vi "Screw.vi"(10 "Clibration 2":T13={"cam 0"={"incident ANGLE COMPENSATION"=[], "dp/B [MeV/C/B]"=[], "charge compensation"=[], "Momentum [MeV/C]"=[], "energyDependence Input"=[], "pixel angle (y)"=[], "dp [MeV/C/] "=[], "angle 2Dfor spectrumj"=[], "dp [MeV/C] 2D"=[], "charge compensation 2D"=[], "Screen&Camera 2"={"Screen Orientation"="Regular", "Screen angle"="Flat", "Lens"=enum."FL1-f8x08", "Calibration (mm/pix)"=1.0}, "ROI info"={"npix-X"=0, "npix-Y"=0, "Left [pix]"=0.0, "Top [pix]"=0.0}, "Y 2D full angle"=[], "calib pixel"={"y1(pixel)"=[], "y2(pixel)"=[], "dp/B [MeV/C/B] (pixel)"=[], "energyDependence Input(pixel)"=[], "bending angle [deg](pixel)"=[], "total path(pixel)"=[], "pixel angle (y)(pixel)"=[], "energy dependence (pixel)"=[], "charge compensation (pixel)"=[], "Momentum [MeV/C](pixel)"=[], "angular compensation(pixel)"=[]}, "2D"={"dp"=[], "chargeCompensation"=[], "angle"=[], "Momentum"=[]}, "UserROI"={"Width"=0.0, "Hight"=0.0, "OffsetX"=0.0, "OffsetY"=0.0}, "final"={"X"=[], "xi"=[], "delta momentum"=0.0, "Y"=[], "yi"=[], "angle (Y)"=[], "delta angle"=0.0, "scale delta angle"=0.0, "intraX"=0.0, "intraY"=0.0, "mask"=[]}, "B[T]"=0.0, "index"=0.0}, "cam 1"={"incident ANGLE COMPENSATION"=[], "dp/B [MeV/C/B]"=[], "charge compensation"=[], "Momentum [MeV/C]"=[], "energyDependence Input"=[], "pixel angle (y)"=[], "dp [MeV/C/] "=[], "angle 2Dfor spectrumj"=[], "dp [MeV/C] 2D"=[], "charge compensation 2D"=[], "Screen&Camera 2"={"Screen Orientation"="Regular", "Screen angle"="Flat", "Lens"=enum."FL1-f8x08", "Calibration (mm/pix)"=1.0}, "ROI info"={"npix-X"=0, "npix-Y"=0, "Left [pix]"=0.0, "Top [pix]"=0.0}, "Y 2D full angle"=[], "calib pixel"={"y1(pixel)"=[], "y2(pixel)"=[], "dp/B [MeV/C/B] (pixel)"=[], "energyDependence Input(pixel)"=[], "bending angle [deg](pixel)"=[], "total path(pixel)"=[], "pixel angle (y)(pixel)"=[], "energy dependence (pixel)"=[], "charge compensation (pixel)"=[], "Momentum [MeV/C](pixel)"=[], "angular compensation(pixel)"=[]}, "2D"={"dp"=[], "chargeCompensation"=[], "angle"=[], "Momentum"=[]}, "UserROI"={"Width"=0.0, "Hight"=0.0, "OffsetX"=0.0, "OffsetY"=0.0}, "final"={"X"=[], "xi"=[], "delta momentum"=0.0, "Y"=[], "yi"=[], "angle (Y)"=[], "delta angle"=0.0, "scale delta angle"=0.0, "intraX"=0.0, "intraY"=0.0, "mask"=[]}, "B[T]"=0.0, "index"=0.0}, "cam 2"={"incident ANGLE COMPENSATION"=[], "dp/B [MeV/C/B]"=[], "charge compensation"=[], "Momentum [MeV/C]"=[], "energyDependence Input"=[], "pixel angle (y)"=[], "dp [MeV/C/] "=[], "angle 2Dfor spectrumj"=[], "dp [MeV/C] 2D"=[], "charge compensation 2D"=[], "Screen&Camera 2"={"Screen Orientation"="Regular", "Screen angle"="Flat", "Lens"=enum."FL1-f8x08", "Calibration (mm/pix)"=1.0}, "ROI info"={"npix-X"=0, "npix-Y"=0, "Left [pix]"=0.0, "Top [pix]"=0.0}, "Y 2D full angle"=[], "calib pixel"={"y1(pixel)"=[], "y2(pixel)"=[], "dp/B [MeV/C/B] (pixel)"=[], "energyDependence Input(pixel)"=[], "bending angle [deg](pixel)"=[], "total path(pixel)"=[], "pixel angle (y)(pixel)"=[], "energy dependence (pixel)"=[], "charge compensation (pixel)"=[], "Momentum [MeV/C](pixel)"=[], "angular compensation(pixel)"=[]}, "2D"={"dp"=[], "chargeCompensation"=[], "angle"=[], "Momentum"=[]}, "UserROI"={"Width"=0.0, "Hight"=0.0, "OffsetX"=0.0, "OffsetY"=0.0}, "final"={"X"=[], "xi"=[], "delta momentum"=0.0, "Y"=[], "yi"=[], "angle (Y)"=[], "delta angle"=0.0, "scale delta angle"=0.0, "intraX"=0.0, "intraY"=0.0, "mask"=[]}, "B[T]"=0.0, "index"=0.0}, "cam 3"={"incident ANGLE COMPENSATION"=[], "dp/B [MeV/C/B]"=[], "charge compensation"=[], "Momentum [MeV/C]"=[], "energyDependence Input"=[], "pixel angle (y)"=[], "dp [MeV/C/] "=[], "angle 2Dfor spectrumj"=[], "dp [MeV/C] 2D"=[], "charge compensation 2D"=[], "Screen&Camera 2"={"Screen Orientation"="Regular", "Screen angle"="Flat", "Lens"=enum."FL1-f8x08", "Calibration (mm/pix)"=1.0}, "ROI info"={"npix-X"=0, "npix-Y"=0, "Left [pix]"=0.0, "Top [pix]"=0.0}, "Y 2D full angle"=[], "calib pixel"={"y1(pixel)"=[], "y2(pixel)"=[], "dp/B [MeV/C/B] (pixel)"=[], "energyDependence Input(pixel)"=[], "bending angle [deg](pixel)"=[], "total path(pixel)"=[], "pixel angle (y)(pixel)"=[], "energy dependence (pixel)"=[], "charge compensation (pixel)"=[], "Momentum [MeV/C](pixel)"=[], "angular compensation(pixel)"=[]}, "2D"={"dp"=[], "chargeCompensation"=[], "angle"=[], "Momentum"=[]}, "UserROI"={"Width"=0.0, "Hight"=0.0, "OffsetX"=0.0, "OffsetY"=0.0}, "final"={"X"=[], "xi"=[], "delta momentum"=0.0, "Y"=[], "yi"=[], "angle (Y)"=[], "delta angle"=0.0, "scale delta angle"=0.0, "intraX"=0.0, "intraY"=0.0, "mask"=[]}, "B[T]"=0.0, "index"=0.0}}, 11 "Settings in":T1) -> (1 "S arrays":T20, 2 "Clibration 2":T13={"cam 0"={"incident ANGLE COMPENSATION"=[], "dp/B [MeV/C/B]"=[], "charge compensation"=[], "Momentum [MeV/C]"=[], "energyDependence Input"=[], "pixel angle (y)"=[], "dp [MeV/C/] "=[], "angle 2Dfor spectrumj"=[], "dp [MeV/C] 2D"=[], "charge compensation 2D"=[], "Screen&Camera 2"={"Screen Orientation"="Regular", "Screen angle"="Flat", "Lens"=enum."FL1-f8x08", "Calibration (mm/pix)"=1.0}, "ROI info"={"npix-X"=0, "npix-Y"=0, "Left [pix]"=0.0, "Top [pix]"=0.0}, "Y 2D full angle"=[], "calib pixel"={"y1(pixel)"=[], "y2(pixel)"=[], "dp/B [MeV/C/B] (pixel)"=[], "energyDependence Input(pixel)"=[], "bending angle [deg](pixel)"=[], "total path(pixel)"=[], "pixel angle (y)(pixel)"=[], "energy dependence (pixel)"=[], "charge compensation (pixel)"=[], "Momentum [MeV/C](pixel)"=[], "angular compensation(pixel)"=[]}, "2D"={"dp"=[], "chargeCompensation"=[], "angle"=[], "Momentum"=[]}, "UserROI"={"Width"=0.0, "Hight"=0.0, "OffsetX"=0.0, "OffsetY"=0.0}, "final"={"X"=[], "xi"=[], "delta momentum"=0.0, "Y"=[], "yi"=[], "angle (Y)"=[], "delta angle"=0.0, "scale delta angle"=0.0, "intraX"=0.0, "intraY"=0.0, "mask"=[]}, "B[T]"=0.0, "index"=0.0}, "cam 1"={"incident ANGLE COMPENSATION"=[], "dp/B [MeV/C/B]"=[], "charge compensation"=[], "Momentum [MeV/C]"=[], "energyDependence Input"=[], "pixel angle (y)"=[], "dp [MeV/C/] "=[], "angle 2Dfor spectrumj"=[], "dp [MeV/C] 2D"=[], "charge compensation 2D"=[], "Screen&Camera 2"={"Screen Orientation"="Regular", "Screen angle"="Flat", "Lens"=enum."FL1-f8x08", "Calibration (mm/pix)"=1.0}, "ROI info"={"npix-X"=0, "npix-Y"=0, "Left [pix]"=0.0, "Top [pix]"=0.0}, "Y 2D full angle"=[], "calib pixel"={"y1(pixel)"=[], "y2(pixel)"=[], "dp/B [MeV/C/B] (pixel)"=[], "energyDependence Input(pixel)"=[], "bending angle [deg](pixel)"=[], "total path(pixel)"=[], "pixel angle (y)(pixel)"=[], "energy dependence (pixel)"=[], "charge compensation (pixel)"=[], "Momentum [MeV/C](pixel)"=[], "angular compensation(pixel)"=[]}, "2D"={"dp"=[], "chargeCompensation"=[], "angle"=[], "Momentum"=[]}, "UserROI"={"Width"=0.0, "Hight"=0.0, "OffsetX"=0.0, "OffsetY"=0.0}, "final"={"X"=[], "xi"=[], "delta momentum"=0.0, "Y"=[], "yi"=[], "angle (Y)"=[], "delta angle"=0.0, "scale delta angle"=0.0, "intraX"=0.0, "intraY"=0.0, "mask"=[]}, "B[T]"=0.0, "index"=0.0}, "cam 2"={"incident ANGLE COMPENSATION"=[], "dp/B [MeV/C/B]"=[], "charge compensation"=[], "Momentum [MeV/C]"=[], "energyDependence Input"=[], "pixel angle (y)"=[], "dp [MeV/C/] "=[], "angle 2Dfor spectrumj"=[], "dp [MeV/C] 2D"=[], "charge compensation 2D"=[], "Screen&Camera 2"={"Screen Orientation"="Regular", "Screen angle"="Flat", "Lens"=enum."FL1-f8x08", "Calibration (mm/pix)"=1.0}, "ROI info"={"npix-X"=0, "npix-Y"=0, "Left [pix]"=0.0, "Top [pix]"=0.0}, "Y 2D full angle"=[], "calib pixel"={"y1(pixel)"=[], "y2(pixel)"=[], "dp/B [MeV/C/B] (pixel)"=[], "energyDependence Input(pixel)"=[], "bending angle [deg](pixel)"=[], "total path(pixel)"=[], "pixel angle (y)(pixel)"=[], "energy dependence (pixel)"=[], "charge compensation (pixel)"=[], "Momentum [MeV/C](pixel)"=[], "angular compensation(pixel)"=[]}, "2D"={"dp"=[], "chargeCompensation"=[], "angle"=[], "Momentum"=[]}, "UserROI"={"Width"=0.0, "Hight"=0.0, "OffsetX"=0.0, "OffsetY"=0.0}, "final"={"X"=[], "xi"=[], "delta momentum"=0.0, "Y"=[], "yi"=[], "angle (Y)"=[], "delta angle"=0.0, "scale delta angle"=0.0, "intraX"=0.0, "intraY"=0.0, "mask"=[]}, "B[T]"=0.0, "index"=0.0}, "cam 3"={"incident ANGLE COMPENSATION"=[], "dp/B [MeV/C/B]"=[], "charge compensation"=[], "Momentum [MeV/C]"=[], "energyDependence Input"=[], "pixel angle (y)"=[], "dp [MeV/C/] "=[], "angle 2Dfor spectrumj"=[], "dp [MeV/C] 2D"=[], "charge compensation 2D"=[], "Screen&Camera 2"={"Screen Orientation"="Regular", "Screen angle"="Flat", "Lens"=enum."FL1-f8x08", "Calibration (mm/pix)"=1.0}, "ROI info"={"npix-X"=0, "npix-Y"=0, "Left [pix]"=0.0, "Top [pix]"=0.0}, "Y 2D full angle"=[], "calib pixel"={"y1(pixel)"=[], "y2(pixel)"=[], "dp/B [MeV/C/B] (pixel)"=[], "energyDependence Input(pixel)"=[], "bending angle [deg](pixel)"=[], "total path(pixel)"=[], "pixel angle (y)(pixel)"=[], "energy dependence (pixel)"=[], "charge compensation (pixel)"=[], "Momentum [MeV/C](pixel)"=[], "angular compensation(pixel)"=[]}, "2D"={"dp"=[], "chargeCompensation"=[], "angle"=[], "Momentum"=[]}, "UserROI"={"Width"=0.0, "Hight"=0.0, "OffsetX"=0.0, "OffsetY"=0.0}, "final"={"X"=[], "xi"=[], "delta momentum"=0.0, "Y"=[], "yi"=[], "angle (Y)"=[], "delta angle"=0.0, "scale delta angle"=0.0, "intraX"=0.0, "intraY"=0.0, "mask"=[]}, "B[T]"=0.0, "index"=0.0}}, 3 "Settings out":T1)   [LabVIEW 2013]
uses:
  Calib_Typdef.ctl
  calib_Sub_Typdef.ctl
  ScreenCam2_TypDEf.ctl
  CamAndObj_TypDEf.ctl
  ROIInfo_TypDef.ctl
  calibPixel.ctl
  2DTypDef.ctl
  CamRoiTypDef.ctl
  finalCalibTypdef.ctl
  settings_TypDef.ctl
  CamSettings_Typdef.ctl
  CamSettingSUB_TypDEf.ctl
  shared/OnOffTypeDef.ctl
  userROI.ctl
  shared/numericVariable_TypeDef.ctl
  SrewMaster_TYpDef.ctl
  srew_TypDEf.ctl
  ScrewSub_Typdef.ctl
  screwstart.ctl
  MagAnalysis_Online.lvclass
  BaseDriver/BaseDriver.lvclass
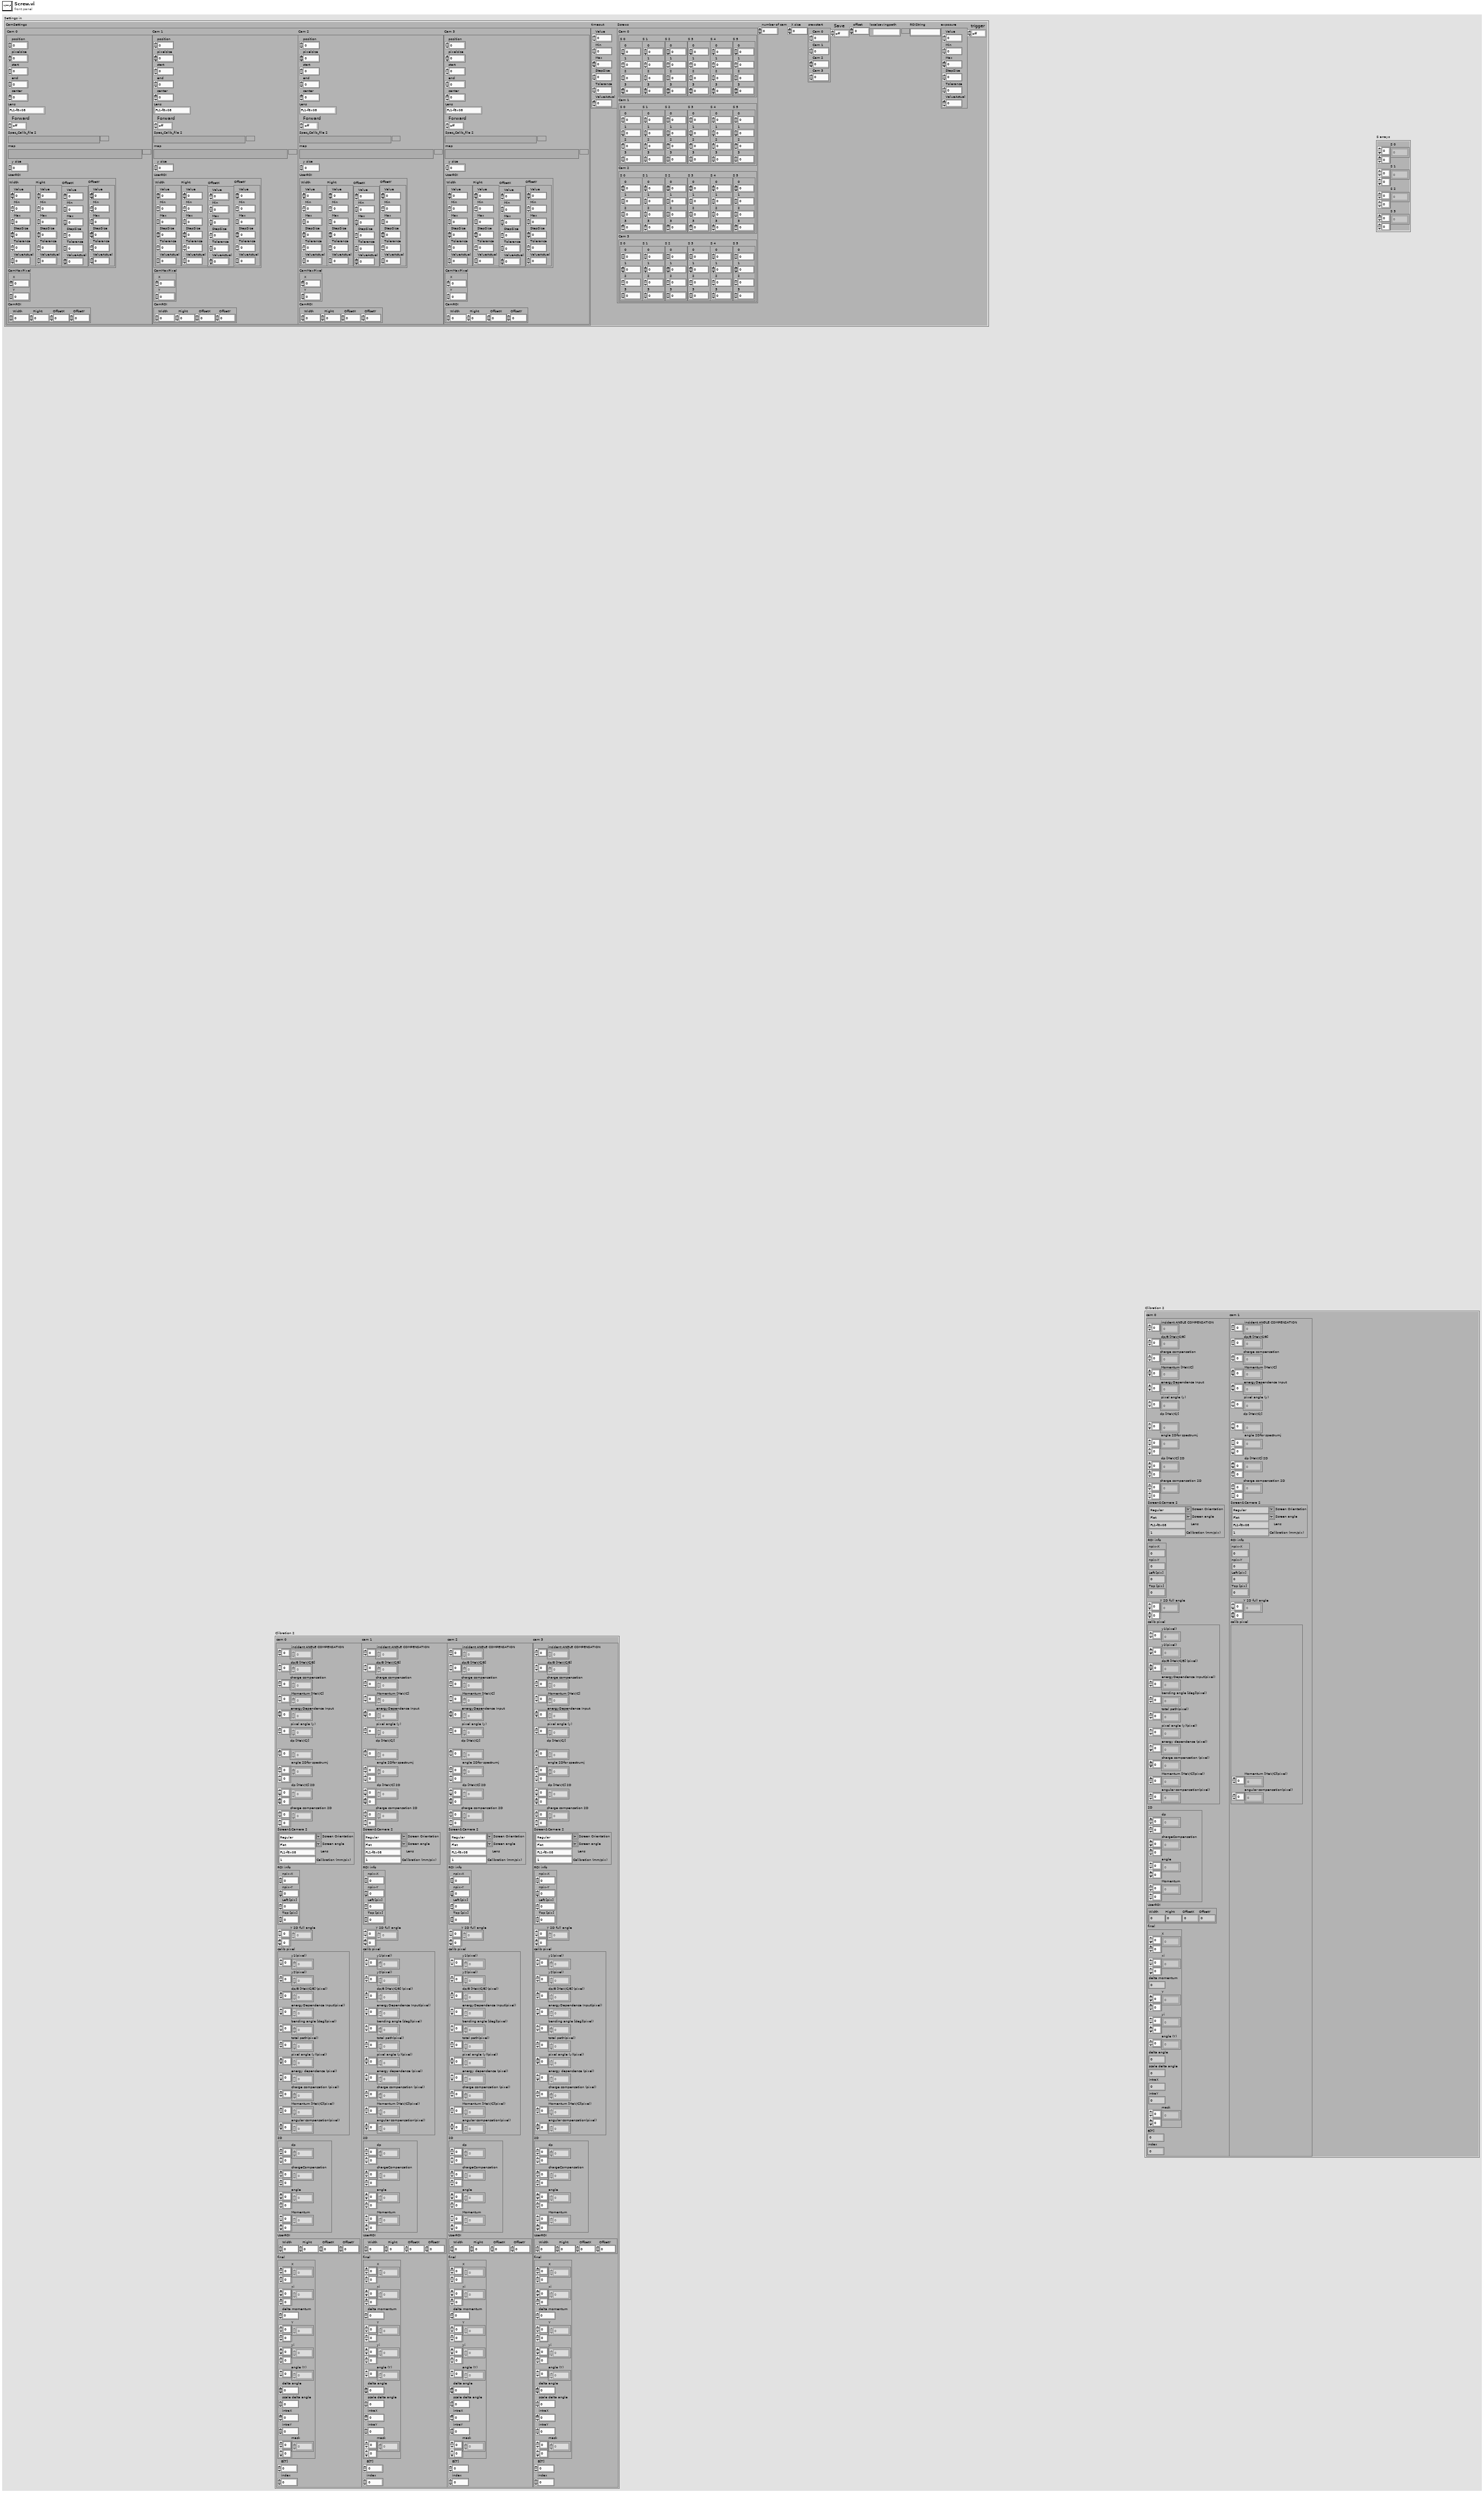
[diagram p1: front panel]
types:
  T1 = typedef "MagAnalysis_Online.lvclass/settings_TypDef.ctl" = cluster{"CamSettings":T2, "timeout":T7, "Screws":T9, "number of cam":dbl, "X size":dbl, "srewstart":T12, "Save":T5, "offset":dbl, "localsavingpath":path, "ROIString":string, "exposure":T7, "trigger":T5}
  T2 = typedef "CamSettings_Typdef.ctl" = cluster{"Cam 0":T3, "Cam 1":T3, "Cam 2":T3, "Cam 3":T3}
  T3 = typedef "CamSettingSUB_TypDEf.ctl" = cluster{"position":dbl, "pixelsize":dbl, "start":dbl, "end":dbl, "center":dbl, "Lens":T4, "Forward":T5, "Spec_Calib_file 2":path, "map":path, "y size":i32, "UserROI":T6, "CamMaxPixel":cluster{"X":i32, "Y":i32}, "CamROI":T8}
  T4 = typedef "CamAndObj_TypDEf.ctl" = enum16{"FL1-f8x08", "FL1-f8x06", "FL1-f8", "ch300-f50", "FL2G-f8", "FL3M14-f8", "FL3M14-f8x08", "FL3M14-f8x08(2x2)"}
  T5 = typedef "OnOffTypeDef.ctl" = enum16{"off", "on"}
  T6 = typedef "userROI.ctl" = cluster{"Width":T7, "Hight":T7, "OffsetX":T7, "OffsetY":T7}
  T7 = typedef "BaseDriver.lvclass/numericVariable_TypeDef.ctl" = cluster{"Value":dbl, "Min":dbl, "Max":dbl, "StepSize":dbl, "Tolerance":dbl, "ValueActual":dbl}
  T8 = typedef "CamRoiTypDef.ctl" = cluster{"Width":dbl, "Hight":dbl, "OffsetX":dbl, "OffsetY":dbl}
  T9 = typedef "SrewMaster_TYpDef.ctl" = cluster{"Cam 0":T10, "Cam 1":T10, "Cam 2":T10, "Cam 3":T10}
  T10 = typedef "srew_TypDEf.ctl" = cluster{"S 0":T11, "S 1":T11, "S 2":T11, "S 3":T11, "S 4":T11, "S 5":T11}
  T11 = typedef "ScrewSub_Typdef.ctl" = cluster{"0":i32, "1":i32, "2":i32, "3":i32}
  T12 = typedef "screwstart.ctl" = cluster{"Cam 0":dbl, "Cam 1":dbl, "Cam 2":dbl, "Cam 3":dbl}
  T13 = typedef "Calib_Typdef.ctl" = cluster{"cam 0":T14, "cam 1":T14, "cam 2":T14, "cam 3":T14}
  T14 = typedef "calib_Sub_Typdef.ctl" = cluster{"incident ANGLE COMPENSATION":dbl[], "dp/B [MeV/C/B]":dbl[], "charge compensation":dbl[], "Momentum [MeV/C]":dbl[], "energyDependence Input":dbl[], "pixel angle (y)":dbl[], "dp [MeV/C/] ":dbl[], "angle 2Dfor spectrumj":dbl[][], "dp [MeV/C] 2D":dbl[][], "charge compensation 2D":dbl[][], "Screen&Camera 2":T15, "ROI info":T16, "Y 2D full angle":dbl[][], "calib pixel":T17, "2D":T18, "UserROI":T8, "final":T19, "B[T]":dbl, "index":dbl}
  T15 = typedef "ScreenCam2_TypDEf.ctl" = cluster{"Screen Orientation":string, "Screen angle":string, "Lens":T4, "Calibration (mm/pix)":dbl}
  T16 = typedef "ROIInfo_TypDef.ctl" = cluster{"npix-X":i32, "npix-Y":i32, "Left [pix]":dbl, "Top [pix]":dbl}
  T17 = typedef "calibPixel.ctl" = cluster{"y1(pixel)":dbl[], "y2(pixel)":dbl[], "dp/B [MeV/C/B] (pixel)":dbl[], "energyDependence Input(pixel)":dbl[], "bending angle [deg](pixel)":dbl[], "total path(pixel)":dbl[], "pixel angle (y)(pixel)":dbl[], "energy dependence (pixel)":dbl[], "charge compensation (pixel)":dbl[], "Momentum [MeV/C](pixel)":dbl[], "angular compensation(pixel)":dbl[]}
  T18 = typedef "2DTypDef.ctl" = cluster{"dp":dbl[][], "chargeCompensation":dbl[][], "angle":dbl[][], "Momentum":dbl[][]}
  T19 = typedef "finalCalibTypdef.ctl" = cluster{"X":dbl[][], "xi":dbl[][], "delta momentum":dbl, "Y":dbl[][], "yi":dbl[][], "angle (Y)":dbl[], "delta angle":dbl, "scale delta angle":dbl, "intraX":dbl, "intraY":dbl, "mask":dbl[][]}
  T20 = cluster{"S 0":i32[][], "S 1":i32[][], "S 2":i32[][], "S 3":i32[][]}
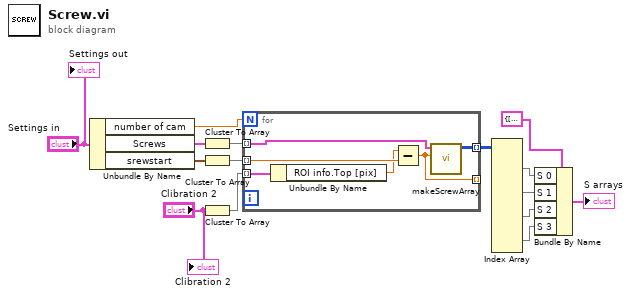
[diagram p0: block diagram]
diagram:
  n1 = Unbundle By Name("Settings in") -> ("number of cam"=w15:dbl, "Screws"=w13:T9, "srewstart"=w14:T12)
  n2 = Cluster To Array(cluster=w13) -> (array=w7:T10[])
  n3 = Cluster To Array(cluster=w14) -> (array=w10:dbl[])
  n4 = Cluster To Array(cluster="Clibration 2") -> (array=w8:T14[])
  n5 = for {
    N: w15 -> [_]
    tunnel: w8 -> [w21] mode=indexing
    tunnel: w7 -> [w20] mode=indexing
    tunnel: [w19] -> w1 mode=indexing
    tunnel: [w17] -> _ mode=indexing
    tunnel: w10 -> [w18] mode=indexing
    n6 = Unbundle By Name(w21) -> ("ROI info.Top [pix]"=w16:dbl)
    n7 = Subtract(x=w16, y=w18) -> (x-y=w17:dbl)
    n8 = call "makeScrewArray.vi"("start"=w17, "Cam 0"=w20) -> ("Array"=w19:i32[][])  [unwired: 9 in]
  }
  n9 = Index Array(array=w1) -> (element #1=w3:i32[][], element #2=w4:i32[][], element #3=w5:i32[][], element #4=w6:i32[][])  [unwired: 12 in]
  n10 = Bundle By Name(cluster=T20 {"S 0"=[], "S 1"=[], "S 2"=[], "S 3"=[]} ("S arrays"), "S 0"=w3, "S 1"=w4, "S 2"=w5, "S 3"=w6) -> (→"S arrays":T20)
  "Clibration 2" <- "Clibration 2"
  "Settings out" <- "Settings in"
